vi "EZ430-Chronos - Read Button (PPT).vi"() -> ()   [LabVIEW 2011, in "LVH-EZ430.lvlib"]
doc: "This example demonstrates how to read the button data from the \nEZ430-Chronos watch in PPT mode."
uses:
  vi.lib/LabVIEW Hacker/LabVIEW Interface for EZ430-Chronos/LVH-EZ430.lvlib
  vi.lib/LabVIEW Hacker/LabVIEW Interface for EZ430-Chronos/Private/Type Defs/EZ430-Chronos Config.ctl
panel:
  out "^":bool
  out "#":bool
  out "*":bool
  in  "EZ430-Chronos Config":T1
  in  "Stop Button":bool
  # "EZ430-Chronos Settings"
  # "Button Status"
  # "EZ430-Chronos Read Button (PPT) Example\n\nThis example demonstrates how to read the button data from the \nEZ430-Chronos watch in PPT mode.\n\nInstructions:\n1. Configure the EZ430-Chronos watch to PPT mode.\n2. Start wireless transmition on the watch.\n3. Select the COM port associated with the EZ430-Chronos USB dongle.\n4. Click the Run Arrow."
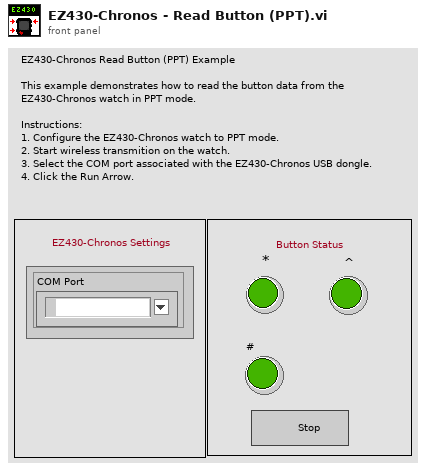
[diagram p1: front panel]
types:
  T1 = typedef "LVH-EZ430.lvlib/EZ430-Chronos Config.ctl" = cluster{"COM Port":refnum<visa-resource-name>}
  T2 = typedef "LVH-EZ430.lvlib/EZ430-Chronos Ref.ctl" = cluster{"COM Port":refnum<visa-resource-name>}
  T3 = typedef "LVH-EZ430.lvlib/Buttons.ctl" = cluster{"*":bool, "#":bool, "^":bool}
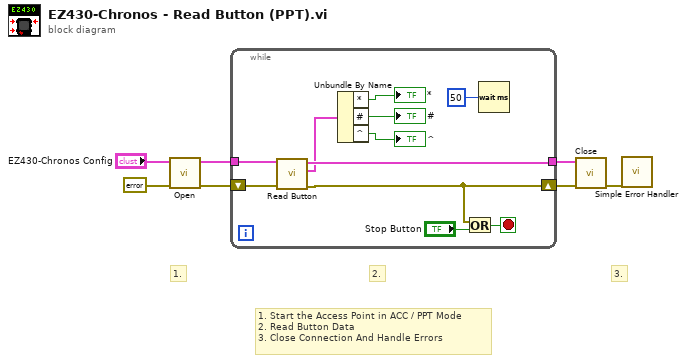
[diagram p0: block diagram]
diagram:
  # "1. Start the Access Point in ACC / PPT Mode\n2. Read Button Data\n3. Close Connection And Handle Errors"
  # "3."
  # "2."
  # "1."
  n1 = call "Open.vi"("Error In"=errorcluster {"status"=FALSE, "code"=0, "source"=""}, "EZ430-Chronos Config"="EZ430-Chronos Config") -> ("Error Out"=w2:errorcluster, "EZ430-Chronos Ref"=w3:T2)  [unwired: 8 in]
  n2 = while {
    tunnel: w3 -> [w15]
    tunnel: [w13] -> w7
    shift-right: [w12] -> w4
    shift-left: w2 -> [w14]
    stop <- w18 stop-if-true
    n3 = call "Read Button.vi"("Error In"=w14, "EZ430-Chronos Ref"=w15) -> ("Error Out"=w12:errorcluster, "Buttons"=w11:T3, "EZ430-Chronos Config"=w13:T2)  [unwired: 7 in]
    n4 = Unbundle By Name(w11) -> ("*"=→"*":bool, "#"=→"#":bool, "^"=→"^":bool)
    n5 = Or(x=w12, y="Stop Button") -> (x .or. y?=w18:bool)
    n6 = Wait (ms)(milliseconds to wait=u32 50) -> ()  [unwired: 1 out]
  }
  n7 = call "Close.vi"("Error In"=w4, "EZ430-Chronos Config"=w7) -> ("Error Out"=w1:errorcluster)  [unwired: 9 in]
  n8 = call <vilib>:"Simple Error Handler.vi"("error in (no error)"=w1) -> ()  [unwired: 4 in, 5 out]
